vi "Get Name.vi"(8 "error in (no error)":errorcluster, 11 "DD Child A in":refnum<class "DD Child A.lvclass">) -> (0 "error out":errorcluster, 2 "name":string, 3 "DD Child A out":refnum<class "DD Child A.lvclass">)   [LabVIEW 2016, in "DD Child A.lvclass"]
uses:
  DD Child A.lvclass
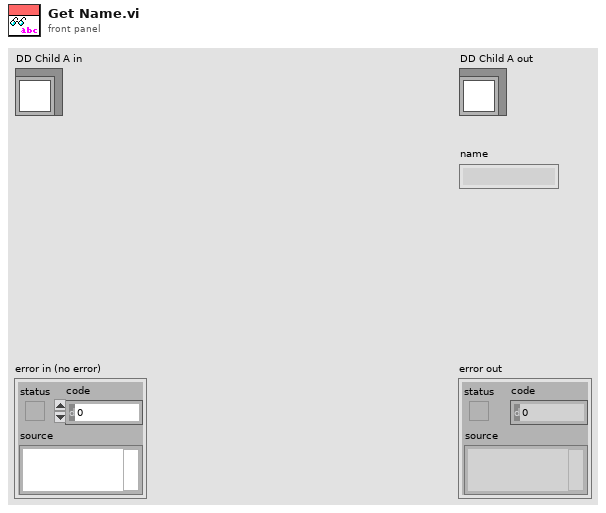
[diagram p1: front panel]
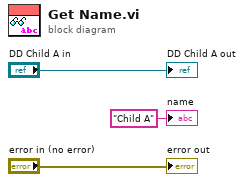
[diagram p0: block diagram]
diagram:
  "error out" <- "error in (no error)"
  "DD Child A out" <- "DD Child A in"
  "name" <- "Child A" ("name")
